vi "Dialogo prosegui collaudo.vi"() -> (2 "PROSEGUI NEW ?":bool)   [LabVIEW 2019]
panel:
  in  "PROSEGUI NEW":bool
  in  "PROSEGUI":bool
  # "MODALITA' PROSEGUI COLLAUDO"
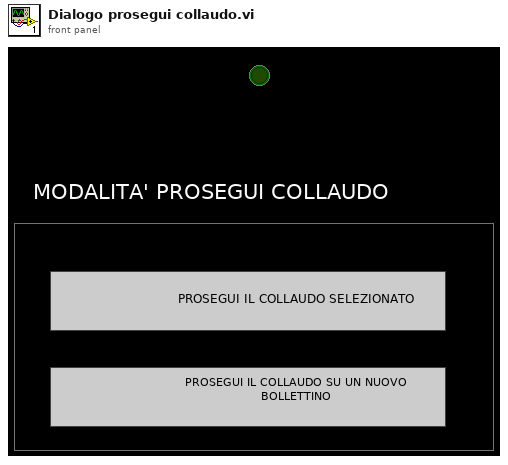
[diagram p1: front panel]
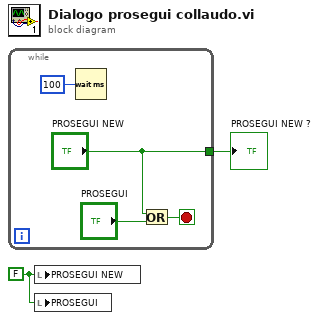
[diagram p0: block diagram]
diagram:
  w2 = FALSE ("PROSEGUI NEW")
  n1 = while {
    tunnel: ["PROSEGUI NEW"] -> w1
    stop <- w4 stop-if-true
    n2 = Wait (ms)(milliseconds to wait=u32 100) -> ()  [unwired: 1 out]
    n3 = Or(x="PROSEGUI NEW", y="PROSEGUI") -> (x .or. y?=w4:bool)
  }
  "PROSEGUI NEW ?" <- w1
  n4 = local write "PROSEGUI NEW"(w2) -> ()
  n5 = local write "PROSEGUI"(w2) -> ()
